vi "Get All Case and Event Frames.vi"(8 "error in (no error)":errorcluster, 11 "JKI SM in":refnum<class "JKI SM.lvclass">) -> (0 "error out":errorcluster, 1 "Event Structure Visible?":bool, 2 "Frame Names":string[](array[string]), 3 "Frames[]":refnum<vi>[](array[refnum]), 4 "Visible Frame Index":i32, 5 "Visible Frame":refnum<vi>, 6 "Visible Frame Name":string, 7 "Num Event Frames":i32, 9 "Event Frame Index":i32)   [LabVIEW 2020]
uses:
  JKI State Machine API/source/JKI SM/JKI SM.lvclass
  JKI State Machine API/source/JKI SM/JKI SM.lvclass/JKI SM.ctl
  <userlib>/_OpenG.lib/string/string.llb/openg_string.lvlib
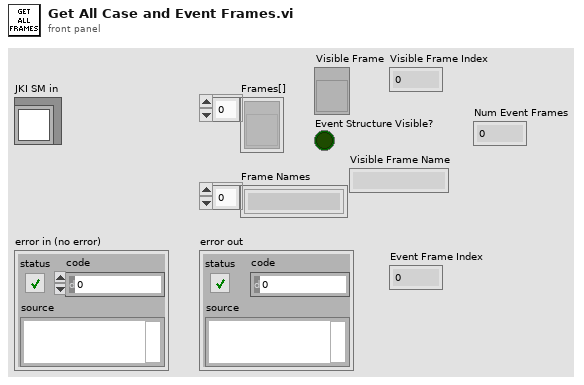
[diagram p1: front panel]
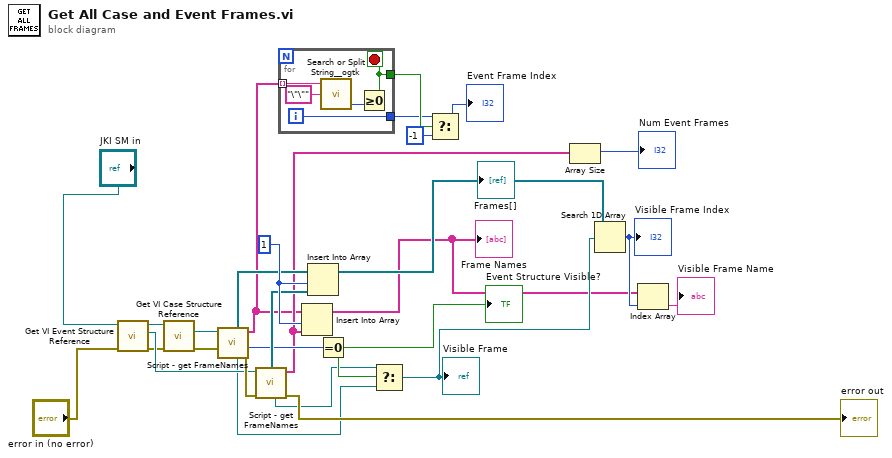
[diagram p0: block diagram]
diagram:
  w23 = 1 ("index")
  n1 = call "Get VI Event Structure Reference.vi"("error in (no error)"="error in (no error)", "JKI SM in"="JKI SM in") -> ("error out"=w17:errorcluster, "Event Structure ref"=w19:refnum<vi>, "JKI SM out"=w24:refnum<class "JKI SM.lvclass">)  [unwired: 7 in]
  n2 = call "Get VI Case Structure Reference.vi"("error in (no error)"=w17, "JKI SM in"=w24) -> ("error out"=w25:errorcluster, "Case Structure ref"=w18:refnum<vi>)  [unwired: 7 in, 1 out]
  n3 = call "Script - get FrameNames.vi"("error in"=w25, "StructRef"=w18) -> ("error out"=w20:errorcluster, "Visible Frame Index"=w16:u32, "Frame Names"=w5:string[], "Visible Frame"=w13:refnum<vi>, "Frames[]"=w22:refnum<vi>[])  [unwired: 4 in, 1 out]
  n4 = call "Script - get FrameNames.vi"("error in"=w20, "StructRef"=w19) -> ("error out"=→"error out":errorcluster, "Frame Names"=w7:string[], "Visible Frame"=w14:refnum<vi>, "Frames[]"=w21:refnum<vi>[])  [unwired: 4 in, 2 out]
  n5 = for {
    tunnel: w5 -> [w33] mode=indexing
    tunnel: [w29] -> w4
    tunnel: [w30] -> w3
    i -> [w30]
    stop <- w29 stop-if-true
    n6 = call <userlib>:"Search or Split String__ogtk.vi"("search string/char (-)"="\"\"", "string"=w33) -> ("offset after match"=w31:i32)  [unwired: 1 in, 2 out]
    n7 = Greater Or Equal To 0?(x=w31) -> (x >= 0?=w29:bool)
  }
  n8 = Insert Into Array(array=w5, index=w23, new element=w7) -> (w9:string[])
  "Frame Names" <- w9
  n9 = Insert Into Array(array=w22, index=w23, new element=w21) -> (w12:refnum<vi>[])
  "Frames[]" <- w12
  n10 = Equal To 0?(x=w16) -> (x = 0?=w15:bool)
  "Event Structure Visible?" <- w15
  n11 = Select(t=w14, s=w15, f=w13) -> (s? t:f=w11:refnum<vi>)
  "Visible Frame" <- w11
  n12 = Select(t=w3, s=w4, f=-1) -> (s? t:f=→"Event Frame Index":i32)
  n13 = Array Size(array=w7) -> (size(s)=→"Num Event Frames":i32)
  n14 = Search 1D Array(1D array=w12, element=w11) -> (index of element=w10:i32)  [unwired: 1 in]
  "Visible Frame Index" <- w10
  n15 = Index Array(array=w9, index=w10) -> (element=→"Visible Frame Name":string)
